vi "AutoMapCalcDist.vi"(8 "Y2":dbl format="%#_13g", 9 "X2":dbl format="%#_13g", 10 "Y1":dbl format="%#_13g", 11 "X1":dbl format="%#_13g") -> (2 "Distance":dbl)   [LabVIEW 2014]
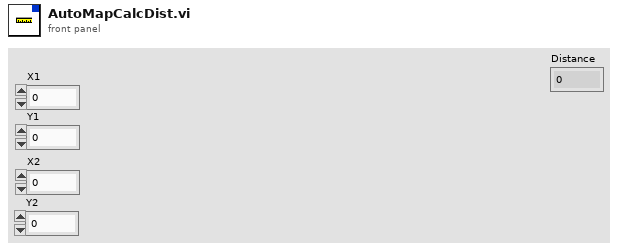
[diagram p1: front panel]
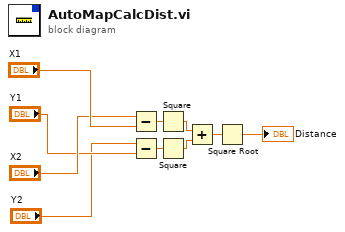
[diagram p0: block diagram]
diagram:
  n1 = Subtract(x="X2", y="X1") -> (x-y=w10:dbl)
  n2 = Subtract(x="Y2", y="Y1") -> (x-y=w9:dbl)
  n3 = Square(x=w10) -> (x^2=w7:dbl)
  n4 = Square(x=w9) -> (x^2=w8:dbl)
  n5 = Add(x=w7, y=w8) -> (x+y=w6:dbl)
  n6 = Square Root(x=w6) -> (sqrt(x)=→"Distance":dbl)
